vi "construct.vi"(8 "error in (no error)":errorcluster, 9 "configuration name":string, 10 "load config file?":bool=TRUE, 11 "YK090623DAQmxAnalogDetector in":refnum<class "DetectorYK090623DAQmxAnalog.lvclass">) -> (0 "error out":errorcluster, 3 "YK090623DAQmxAnalogDetector out":refnum<class "DetectorYK090623DAQmxAnalog.lvclass">)   [LabVIEW 2010, in "DetectorYK090623DAQmxAnalog.lvclass"]
uses:
  DetectorYK090623DAQmxAnalog.lvclass
  GenericDetector/GenericDetector/GenericDetector.lvclass
  DetectorYK090623DAQmxAnalog.lvclass/DetectorYK090623DAQmxAnalog.ctl
  AnalogOut/AnalogOutDL101207DAQmx/AnalogOutDL101207DAQmx/AnalogOutDL101207DAQmx.lvclass
  common/classes/ErrorController/ErrorController/class_data.vi
  common/classes/ErrorController/ErrorController/ErrorController.lvclass
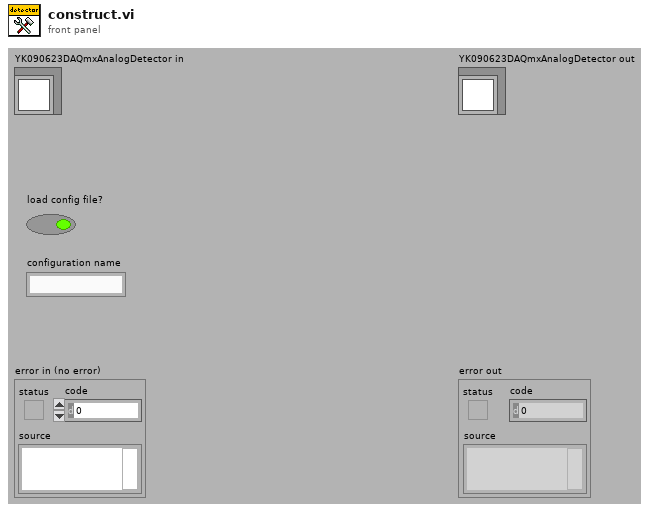
[diagram p1: front panel]
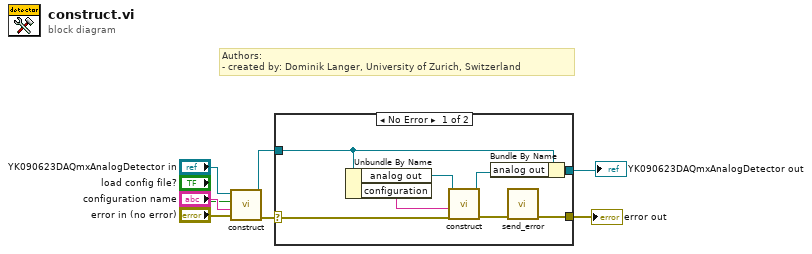
[diagram p0: block diagram]
diagram:
  # "Authors: \n- created by: Dominik Langer, University of Zurich, Switzerland"
  n1 = call-parent "construct.vi"("error in (no error)"="error in (no error)", "configuration name"="configuration name", "load config file?"="load config file?", "GenericPlugin in"="YK090623DAQmxAnalogDetector in") -> ("error out"=w4:errorcluster, "GenericPlugin out"=w3:refnum<class "DetectorYK090623DAQmxAnalog.lvclass">)  [unwired: 6 out]
  n2 = case shown="No Error" w4 {
    selector: w4 -> [w16 w17]
    tunnel: w3 -> [w13 w18]
    tunnel: [w12 w18] -> w2
    tunnel: [w9 w17] -> w1
    frame No Error {
      n3 = Unbundle By Name(w13) -> ("analog out"=w15:refnum<class "AnalogOutDL101207DAQmx.lvclass">, "configuration"=w11:string)
      n4 = call-dynamic "construct.vi"("error in (no error)"=w16, "configuration name"=w11, "GenericPlugin in"=w15) -> ("error out"=w10:errorcluster, "GenericPlugin out"=w14:refnum<class "AnalogOutDL101207DAQmx.lvclass">)  [unwired: 1 in, 6 out]
      n5 = Bundle By Name(cluster=w13, "analog out"=w14) -> (w12:refnum<class "DetectorYK090623DAQmxAnalog.lvclass">)
      n6 = call "send_error.vi"("error in (no error)"=w10) -> ("error out"=w9:errorcluster)  [unwired: 10 in]
    }
    frame Error {
    }
  }
  "error out" <- w1
  "YK090623DAQmxAnalogDetector out" <- w2
